vi "insertXMLNode.vi"(8 "error in (no error)":errorcluster, 9 "xmlString":string, 10 "xmlPath":string, 11 "xmlNode in":refnum<class "xmlNode.lvclass">) -> (0 "error out":errorcluster, 2 "newXMLNode":refnum<class "xmlNode.lvclass">, 3 "xmlNode out":refnum<class "xmlNode.lvclass">)   [LabVIEW 2011, in "Tools.lvlib" / "xml.lvlib" / "xmlNode.lvclass"]
doc: "Insert an xml node into the xml structure"
uses:
  xmlNode.lvclass
  XmlParser.lvclass
panel:
  out "String":string
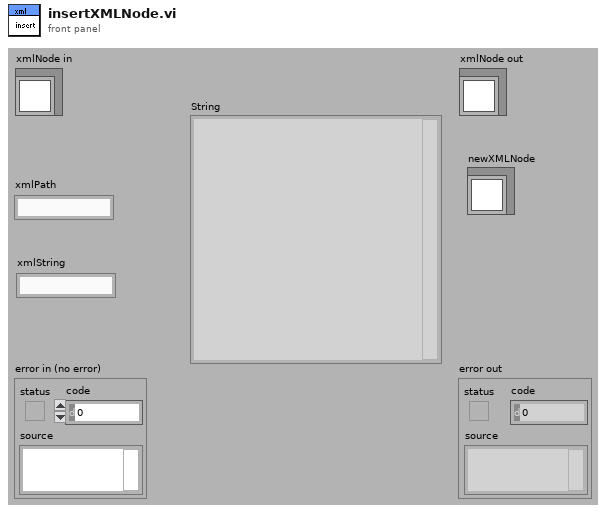
[diagram p1: front panel]
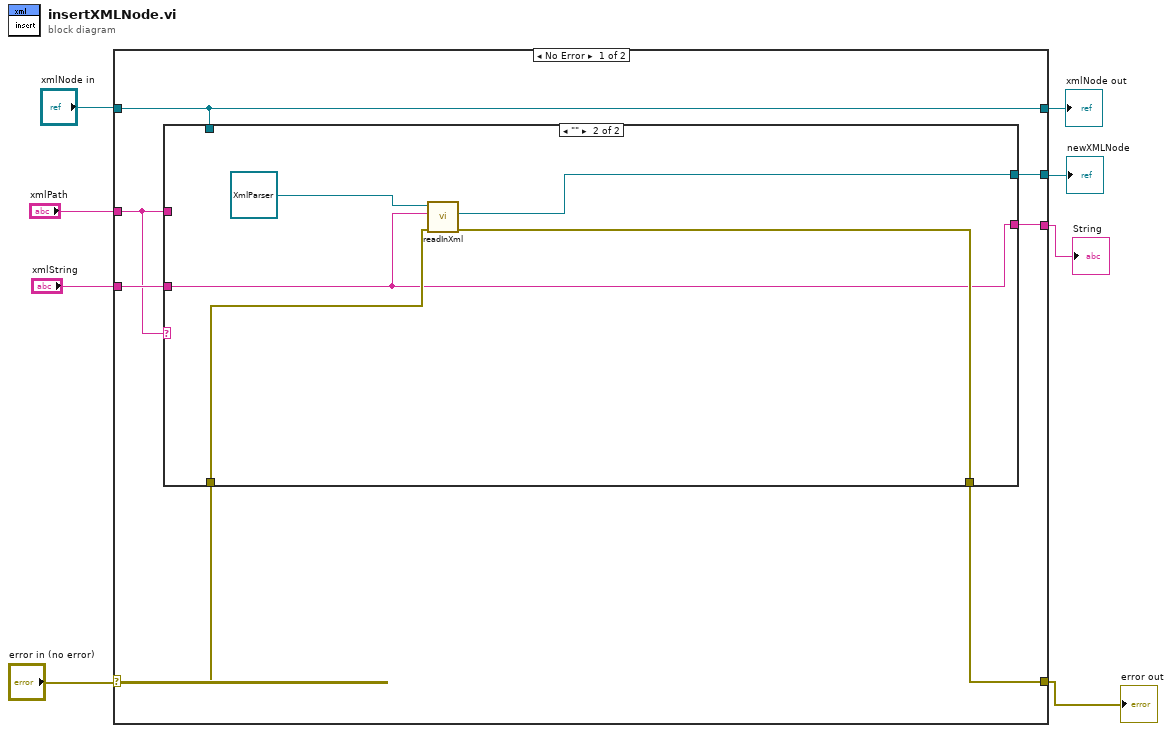
[diagram p0: block diagram]
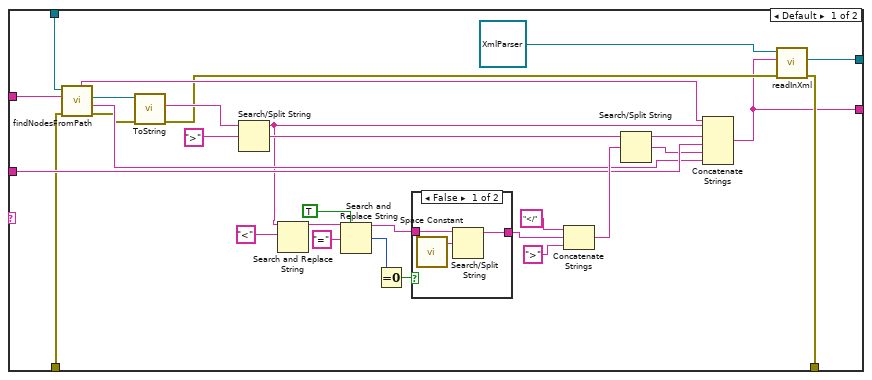
[diagram p2: hidden frame]
diagram:
  n1 = case shown="No Error" "error in (no error)" {
    selector: "error in (no error)" -> [w13 w56]
    tunnel: [w12 w56] -> w7
    tunnel: [w15 w55] -> w5
    tunnel: "xmlNode in" -> [w15 w55]
    tunnel: "xmlPath" -> [w9 _]
    tunnel: "xmlString" -> [w14 _]
    tunnel: [w11 _] -> w2
    tunnel: [w10 _] -> w1
    frame No Error {
      n2 = case shown="\"\"" w9 {
        tunnel: w15 -> [w45 _]
        tunnel: w9 -> [w37 _]
        tunnel: w14 -> [w29 w51]
        tunnel: w13 -> [w22 w53]
        tunnel: [w21 w52] -> w12
        tunnel: [w20 w50] -> w11
        tunnel: [w16 w51] -> w10
        frame Default {
          w42 = "="
          n3 = call "findNodesFromPath.vi"("error in (no error)"=w22, "searchInElement"=w37, "xmlNode in"=w45) -> ("error out"=w23:errorcluster, "rest of xml"=w26:string, "xmlNode"=w44:refnum<class "xmlNode.lvclass">, "xml before"=w28:string)  [unwired: 4 in, 1 out]
          n4 = call-dynamic "ToString.vi"("error in (no error)"=w23, "xmlNode in"=w44) -> ("error out"=w24:errorcluster, "xml"=w43:string)  [unwired: 7 in, 1 out]
          n5 = Search/Split String(string=w43, search string/char (-)=">") -> (substring before match=w19:string, match + rest of string=w35:string)  [unwired: 1 in, 1 out]
          n6 = Search and Replace String(input string=w19, search string="<") -> (result string=w17:string)  [unwired: 6 in, 3 out]
          n7 = Search and Replace String(replace all?=TRUE, input string=w17, search string=w42, replace string=w42) -> (result string=w39:string, number of replacements=w41:i32)  [unwired: 4 in, 2 out]
          n8 = Equal To 0?(x=w41) -> (x = 0?=w40:bool)
          n9 = case shown="False" w40 {
            tunnel: w39 -> [w48 w49]
            tunnel: [w46 w49] -> w33
            frame False {
              n10 = call <vilib>:"Space Constant.vi"() -> ("String"=w47:string)
              n11 = Search/Split String(string=w48, search string/char (-)=w47) -> (substring before match=w46:string)  [unwired: 1 in, 2 out]
            }
            frame True {
            }
          }
          n12 = Concatenate Strings("</", w33, ">") -> (w31:string)
          n13 = Search/Split String(string=w35, search string/char (-)=w31) -> (substring before match=w30:string, match + rest of string=w27:string)  [unwired: 1 in, 1 out]
          n14 = Concatenate Strings(w28, w19, w30, w29, w27, w26) -> (w16:string)
          n15 = call "readInXml.vi"("error in (no error)"=w24, "xmlString"=w16, "XmlParser in"=refnum<class "XmlParser.lvclass"> refnum ("Tools.lvlib:XmlParser.lvclass")) -> ("error out"=w21:errorcluster, "xmlNode"=w20:refnum<class "xmlNode.lvclass">)  [unwired: 6 in, 1 out]
        }
        frame "" {
          n16 = call "readInXml.vi"("error in (no error)"=w53, "xmlString"=w51, "XmlParser in"=refnum<class "XmlParser.lvclass"> refnum ("Tools.lvlib:xml.lvlib:XmlParser.lvclass")) -> ("error out"=w52:errorcluster, "xmlNode"=w50:refnum<class "xmlNode.lvclass">)  [unwired: 6 in, 1 out]
        }
      }
    }
    frame Error {
    }
  }
  "error out" <- w7
  "xmlNode out" <- w5
  "newXMLNode" <- w2
  "String" <- w1
